vi "close_data_log.vi"(8 "error in (no error)":errorcluster, 11 "tt20_logger in":refnum<class "tt20_logger.lvclass">) -> (0 "error out":errorcluster, 3 "tt20_logger out":refnum<class "tt20_logger.lvclass">)   [LabVIEW 2015, in "tt20_logger.lvclass"]
uses:
  tt20_logger.lvclass
  tt20_logger.lvclass/tt20_logger.ctl
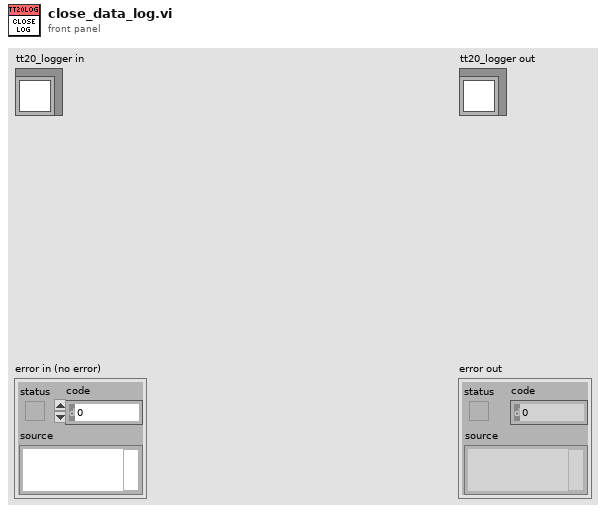
[diagram p1: front panel]
types:
  T1 = typedef "HDF5 Ref.ctl" = refnum<k1>
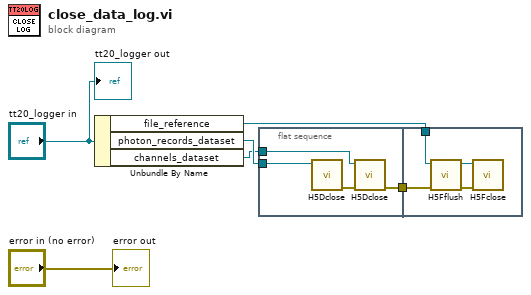
[diagram p0: block diagram]
diagram:
  n1 = Unbundle By Name("tt20_logger in") -> ("file_reference"=w4:T1, "photon_records_dataset"=w3:T1, "channels_dataset"=w2:T1)
  n2 = flat-sequence {
    tunnel: w3 -> [w10]
    tunnel: w2 -> [w9]
    tunnel: [w7] -> w1
    tunnel: w4 -> [w13]
    tunnel: w1 -> [w12]
    frame #0 {
      n3 = call <vilib>:"H5Dclose.vi"("HDF5 Dataset Ref"=w10) -> ("error out"=w8:errorcluster)  [unwired: 8 in]
      n4 = call <vilib>:"H5Dclose.vi"("error in (no error)"=w8, "HDF5 Dataset Ref"=w9) -> ("error out"=w7:errorcluster)  [unwired: 7 in]
    }
    frame #1 {
      n5 = call <vilib>:"H5Fflush.vi"("error in (no error)"=w12, "HDF5 Ref"=w13) -> ("error out"=w11:errorcluster, "HDF5 Ref out"=w14:T1)  [unwired: 6 in]
      n6 = call <vilib>:"H5Fclose.vi"("error in (no error)"=w11, "HDF5 Ref"=w14) -> ()  [unwired: 7 in, 1 out]
    }
  }
  "error out" <- "error in (no error)"
  "tt20_logger out" <- "tt20_logger in"
